vi "irsensorexample.vi"(11 "Read Voltage":dbl) -> (3 "Distance in centimeters":dbl)   [LabVIEW 2015]
uses:
  <vilib>/Analysis/NI_AALPro.lvlib
panel:
  # "Setup: The top recessed frame has 3 fields, for the purpose of this example the Cutoff Frequency is set to 10 Hz, this frequency is used by the low pass filter to remove any stray spike that might occur.\nThe Sample Rate is the rate at which the each of the Number of Samples to Read are being read in at. The Number of Samples is the number of samples the myDAQ is told to acquire before returning data.\n\nAverage of Voltage Samples: This indicator shows the average of the samples being read in.\n\nVoltage Samples Over Time: Displays each set of sample's average value over time.\n\nRaw Data from myDAQ: Displays the sample set that is being retrieved.\n\nFiltered Signal from myDAQ: Displays the sample set after having the low pass filter applied\n\nDistance in centimeters: Displays the distance obtained after sending the average voltage into spline interpolation. The limits are set to 15cm to 150cm which are accurate limits of the infrared sensor."
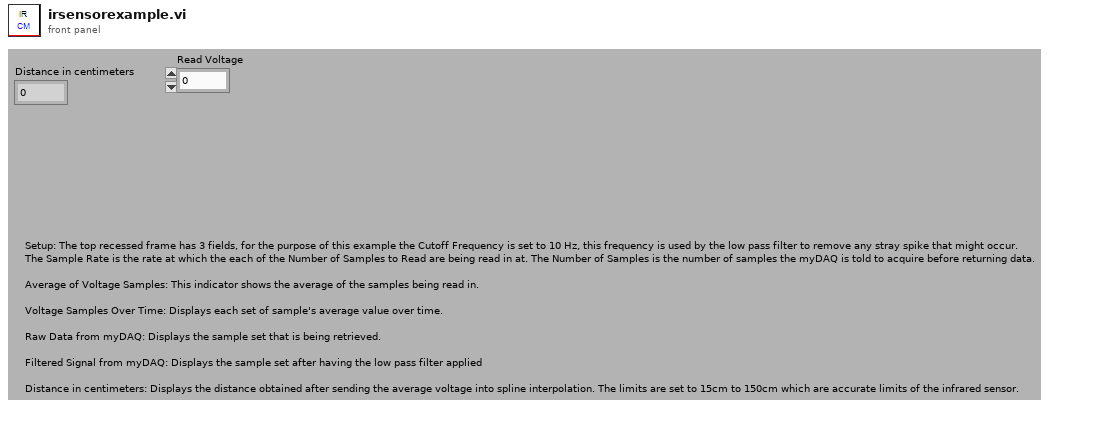
[diagram p1: front panel]
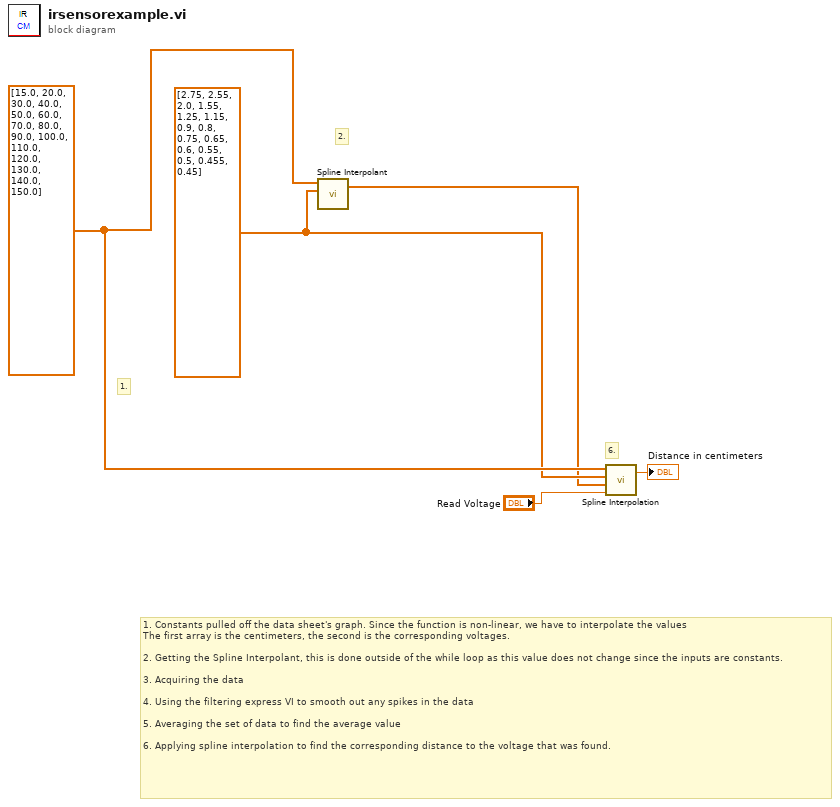
[diagram p0: block diagram]
diagram:
  w5 = dbl[] [15.0, 20.0, 30.0, 40.0, 50.0, 60.0, 70.0, 80.0, 90.0, 100.0, 110.0, 120.0, 130.0, 140.0, 150.0] ("Y")
  w4 = dbl[] [2.75, 2.55, 2.0, 1.55, 1.25, 1.15, 0.9, 0.8, 0.75, 0.65, 0.6, 0.55, 0.5, 0.455, 0.45] ("Y")
  # "6."
  # "2."
  # "1."
  # "1. Constants pulled off the data sheet's graph. Since the function is non-linear, we have to interpolate the values\nThe first array is the centimeters, the second is the corresponding voltages.\n\n2. Getting the Spline Interpolant, this is done outside of the while loop as this value does not change since the inputs are constants.\n\n3. Acquiring the data\n\n4. Using the filtering express VI to smooth out any spikes in the data\n\n5. Averaging the set of data to find the average value\n\n6. Applying spline interpolation to find the corresponding distance to the voltage that was found."
  n1 = call <vilib>:"Spline Interpolant.vi"("X"=w4, "Y"=w5) -> ("Interpolant"=w3:dbl[])  [unwired: 2 in, 1 out]
  n2 = call <vilib>:"Spline Interpolation.vi"("x value"="Read Voltage", "Interpolant"=w3, "X"=w4, "Y"=w5) -> ("interpolation value"=→"Distance in centimeters":dbl)  [unwired: 1 out]
